vi "Noise_Box_Temps.vi"() -> ()   [LabVIEW 2009]
panel:
  in  "stop":bool
  out "InsideBox":dbl(graph)
  out "Outside Box":dbl(graph)
  out "String_Temp_NoiseBoxes":string
  out "error out":errorcluster
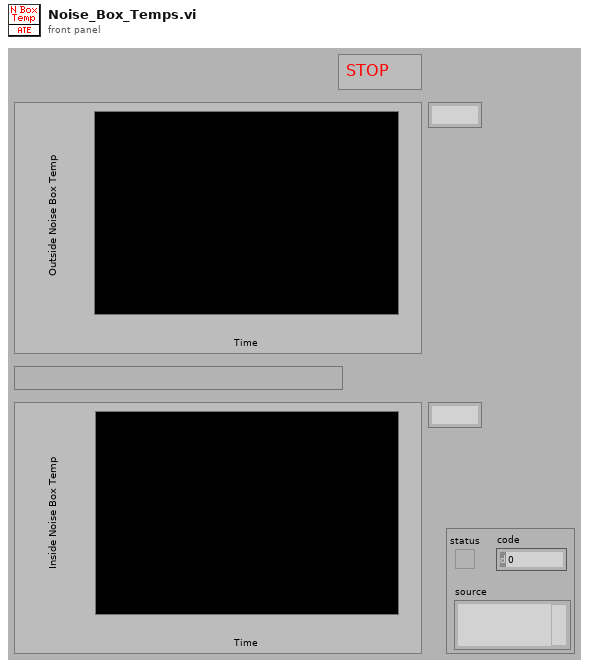
[diagram p1: front panel]
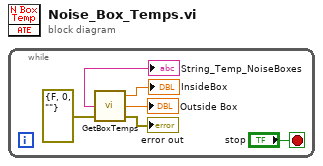
[diagram p0: block diagram]
diagram:
  n1 = while {
    stop <- "stop" stop-if-true
    n2 = call "GetBoxTemps.vi"("error in (no error)"=errorcluster {"status"=FALSE, "code"=0, "source"=""}) -> ("error out"=→"error out":errorcluster, "Outside Box"=→"Outside Box":dbl, "InsideBox"=→"InsideBox":dbl, "String_Temp_NoiseBoxes"=→"String_Temp_NoiseBoxes":string)  [unwired: 1 in]
  }
